vi "DHE_Macro.vi"(8 "error in (no error)":errorcluster, 10 "macro":string, 11 "fd":i32) -> (0 "error out":errorcluster, 2 "response":string)   [LabVIEW 2016]
panel:
  in  "refnum":refnum<vi>
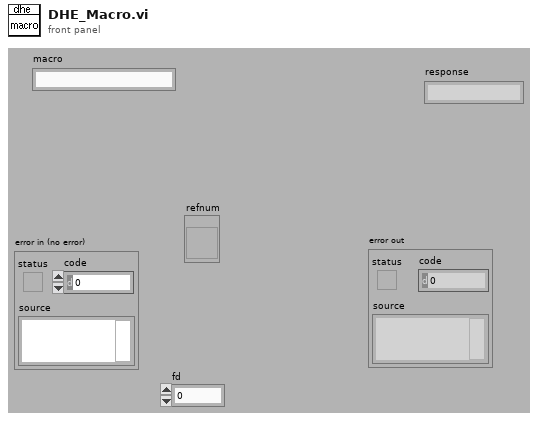
[diagram p1: front panel]
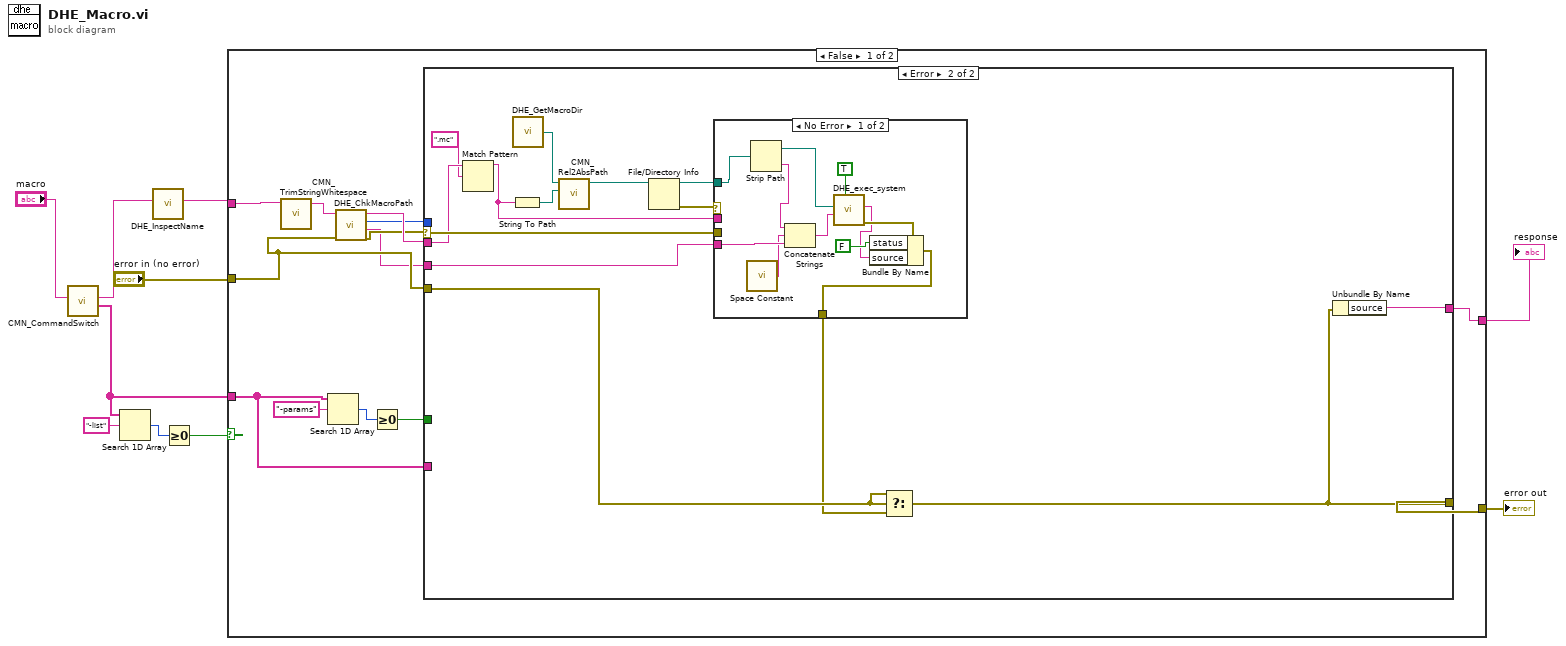
[diagram p0: block diagram]
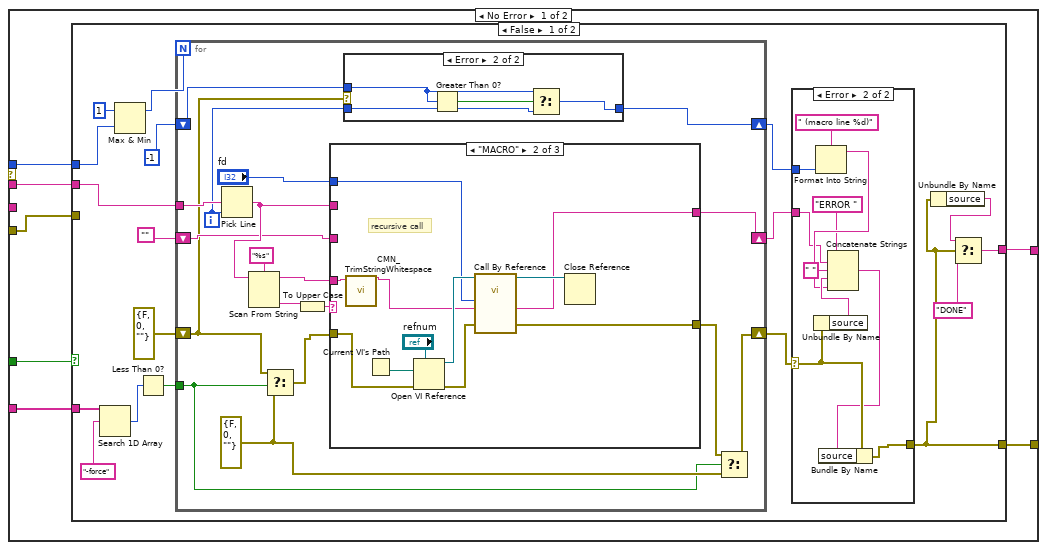
[diagram p2: hidden frame]
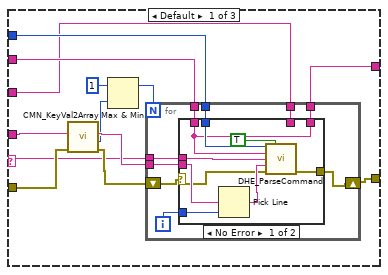
[diagram p4: hidden frame]
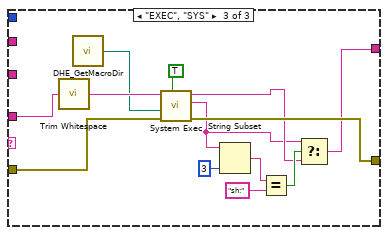
[diagram p6: hidden frame]
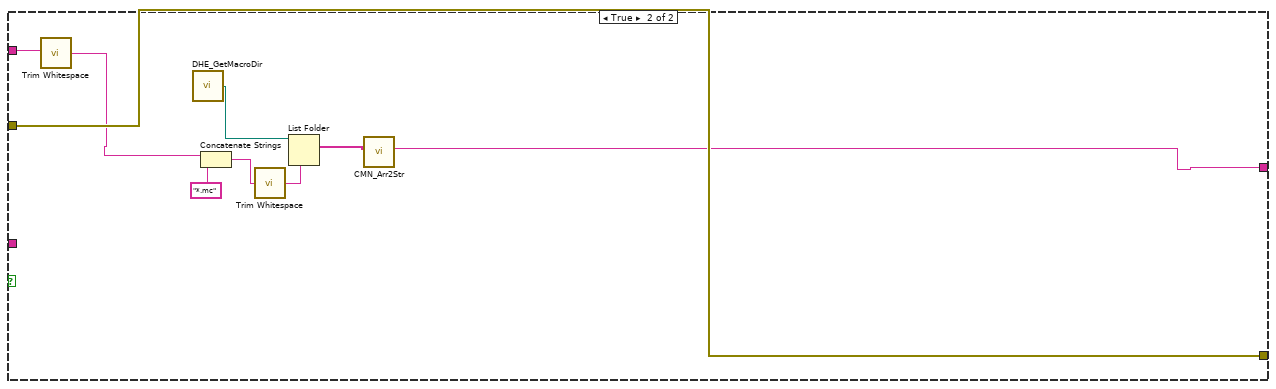
[diagram p10: hidden frame]
diagram:
  n1 = call "CMN_CommandSwitch.vi"("command in"="macro") -> ("swhitches"=w3:string[], "command out"=w2:string)  [unwired: 1 in, 8 out]
  n2 = Search 1D Array(1D array=w3, element="-list") -> (index of element=w8:i32)  [unwired: 1 out]
  n3 = call "DHE_InspectName.vi"("name in"=w2) -> ("name out"=w1:string)  [unwired: 10 out]
  n4 = Greater Or Equal To 0?(x=w8) -> (x >= 0?=w6:bool)
  n5 = case shown="False" w6 {
    tunnel: [w18 w174] -> w10
    tunnel: w1 -> [w20 w169]
    tunnel: "error in (no error)" -> [w19 w174]
    tunnel: [w14 w173] -> w5
    tunnel: w3 -> [w13 _]
    frame False {
      n6 = call "CMN_TrimStringWhitespace.vi"("string"=w20) -> ("trimmed string"=w12:string)  [unwired: 1 in, 8 out]
      n7 = Search 1D Array(1D array=w13, element="-params") -> (index of element=w16:i32)  [unwired: 1 out]
      n8 = call "DHE_ChkMacroPath.vi"("error in (no error)"=w19, "macro name"=w12) -> ("error out"=w22:errorcluster, "args"=w11:string, "number of lines"=w21:i32, "macro out"=w23:string)  [unwired: 6 out]
      n9 = Greater Or Equal To 0?(x=w16) -> (x >= 0?=w15:bool)
      n10 = case shown="Error" w22 {
        selector: w22 -> [_ w147]
        tunnel: [w27 w154] -> w18
        tunnel: w23 -> [w29 w144]
        tunnel: w21 -> [w30 _]
        tunnel: w19 -> [w25 w155]
        tunnel: w15 -> [w28 _]
        tunnel: [w26 w153] -> w14
        tunnel: w13 -> [w24 _]
        tunnel: w11 -> [_ w145]
        frame No Error {
          n11 = case shown="False" w28 {
            tunnel: w30 -> [w46 _]
            tunnel: w29 -> [w45 w141]
            tunnel: [w38 w140] -> w27
            tunnel: [w37 w141] -> w26
            tunnel: w25 -> [_ w140]
            tunnel: w24 -> [w34 _]
            frame False {
              n12 = Search 1D Array(1D array=w34, element="-force") -> (index of element=w32:i32)  [unwired: 1 out]
              n13 = Max & Min(x=1, y=w46) -> (max(x,y)=w47:i32)  [unwired: 1 out]
              n14 = Less Than 0?(x=w32) -> (x < 0?=w31:bool)
              n15 = for {
                N: w47 -> [_]
                shift-right: [w60] -> w42
                shift-left: errorcluster {"status"=FALSE, "code"=0, "source"=""} ("error out") -> [w65]
                tunnel: w45 -> [w74]
                shift-right: [w72] -> w41
                shift-left: -1 -> [w71]
                shift-right: [w68] -> w36
                shift-left: "" -> [w67]
                tunnel: w31 -> [w61]
                i -> [w73]
                w62 = errorcluster {"status"=FALSE, "code"=0, "source"=""} ("f")
                n16 = Pick Line(multi-line string=w74, line index=w73) -> (output string=w69:string)  [unwired: 1 out]
                n17 = Scan From String(format string="%s", input string=w69) -> (remaining string=w75:string, output 1=w76:string)  [unwired: 2 in, 3 out]
                n18 = Select(t=w65, s=w61, f=w62) -> (s? t:f=w64:errorcluster)
                n19 = To Upper Case(1:w76) -> (0:w66:string)
                n20 = case shown="\"MACRO\"" w66 {
                  selector: w66 -> [w83 _ _]
                  tunnel: w69 -> [w80 _ _]
                  tunnel: w75 -> [w84 w121 w132]
                  tunnel: w64 -> [w85 w114 w133]
                  tunnel: [w82 w116 w134] -> w63
                  tunnel: "fd" -> [w81 w115 _]
                  tunnel: [w79 w111 w124] -> w68
                  tunnel: w67 -> [w78 _ _]
                  frame Default {
                    n21 = call "CMN_KeyVal2Array.vi"("error in (no error)"=w85, "command in"=w84) -> ("error out"=w89:errorcluster, "number of commands"=w88:i32, "commands out"=w90:string)  [unwired: 1 in, 5 out]
                    n22 = Max & Min(x=1, y=w88) -> (max(x,y)=w86:i32)  [unwired: 1 out]
                    n23 = for {
                      N: w86 -> [_]
                      tunnel: w81 -> [w99]
                      tunnel: w80 -> [w98]
                      tunnel: w83 -> [w97]
                      tunnel: w90 -> [w94]
                      shift-right: [w96] -> w82
                      shift-left: w89 -> [w93]
                      tunnel: [w92] -> w79
                      tunnel: w78 -> [w91]
                      i -> [w95]
                      n24 = case shown="No Error" w93 {
                        selector: w93 -> [w102 w110]
                        tunnel: w99 -> [w108 _]
                        tunnel: w98 -> [w101 _]
                        tunnel: w97 -> [w107 _]
                        tunnel: [w106 w110] -> w96
                        tunnel: w95 -> [w105 _]
                        tunnel: w94 -> [w104 _]
                        tunnel: [w101 w109] -> w92
                        tunnel: w91 -> [_ w109]
                        frame No Error {
                          n25 = Pick Line(multi-line string=w104, line index=w105) -> (output string=w103:string)  [unwired: 1 out]
                          n26 = call "DHE_ParseCommand.vi"("fd"=w108, "Log"=TRUE, "command + args"=w101, "command"=w107, "arguments"=w103, "error in"=w102) -> ("error out"=w106:errorcluster)  [unwired: 1 in, 8 out]
                        }
                        frame Error {
                        }
                      }
                    }
                  }
                  frame "MACRO" {
                    # "recursive call"
                    n27 = call "CMN_TrimStringWhitespace.vi"("string"=w121) -> ("trimmed string"=w117:string)  [unwired: 1 in, 8 out]
                    n28 = Current VI's Path() -> (path=w119:path)
                    n29 = Open VI Reference(type specifier VI Refnum (for type only)="refnum", vi path=w119, error in (no error)=w114) -> (vi reference=w118:refnum<vi>, error out=w113:errorcluster)  [unwired: 3 out]
                    n30 = call-by-ref "?"(reference=w118, "error in (no error)"=w113, "macro"=w117, "fd"=w115) -> (reference out=w112:refnum<vi>, "error out"=w116:errorcluster, "response"=w111:string)  [unwired: 8 in, 1 out]
                    n31 = Close Reference(reference=w112) -> ()  [unwired: 1 in, 1 out]
                  }
                  frame "EXEC", "SYS" {
                    n32 = call <vilib>:"Trim Whitespace.vi"("string"=w132) -> ("trimmed string"=w131:string)  [unwired: 1 in]
                    n33 = call "DHE_GetMacroDir.vi"() -> ("DHE_MacroDir"=w129:path)  [unwired: 9 out]
                    n34 = call <vilib>:"System Exec.vi"("wait until completion? (T)"=TRUE, "error in (no error)"=w133, "working directory"=w129, "command line"=w131) -> ("error out"=w134:errorcluster, "standard error"=w122:string, "standard output"=w123:string)  [unwired: 2 in, 3 out]
                    n35 = String Subset(string=w122, length (rest)=3 ("length (rest)")) -> (substring=w125:string)  [unwired: 1 out]
                    n36 = Equal?(x=w125, y="sh:") -> (x = y?=w126:bool)
                    n37 = Select(t=w122, s=w126, f=w123) -> (s? t:f=w124:string)
                  }
                }
                n38 = case shown="Error" w65 {
                  tunnel: w73 -> [_ w137]
                  tunnel: [w135 w136] -> w72
                  tunnel: w71 -> [w135 w138]
                  frame No Error {
                  }
                  frame Error {
                    n39 = Greater Than 0?(x=w138) -> (x > 0?=w139:bool)
                    n40 = Select(t=w138, s=w139, f=w137) -> (s? t:f=w136:i32)
                  }
                }
                n41 = Select(t=w63, s=w61, f=w62) -> (s? t:f=w60:errorcluster)
              }
              n42 = case shown="Error" w42 {
                selector: w42 -> [w49 w58]
                tunnel: [w49 w57] -> w38
                tunnel: w41 -> [_ w55]
                tunnel: w36 -> [_ w51]
                frame No Error {
                }
                frame Error {
                  n43 = Unbundle By Name(w58) -> ("source"=w59:string)
                  n44 = Format Into String(format string=" (macro line %d)", w55) -> (resulting string=w53:string)  [unwired: 2 in, 1 out]
                  n45 = Concatenate Strings("ERROR " ("string"), w51, " " ("string"), w59, w53) -> (w56:string)
                  n46 = Bundle By Name(cluster=w58, "source"=w56) -> (w57:errorcluster)
                }
              }
              n47 = Unbundle By Name(w38) -> ("source"=w39:string)
              n48 = Select(t=w39, s=w38, f="DONE") -> (s? t:f=w37:string)
            }
            frame True {
            }
          }
        }
        frame Error {
          n49 = Match Pattern(string=w144, regular expression=".mc") -> (before substring=w142:string)  [unwired: 1 in, 3 out]
          n50 = String To Path(string=w142) -> (path=w149:path)
          n51 = call "DHE_GetMacroDir.vi"() -> ("DHE_MacroDir"=w150:path)  [unwired: 9 out]
          n52 = call "CMN_Rel2AbsPath.vi"("test path"=w149, "absolute path"=w150) -> ("output path"=w151:path)  [unwired: 1 in, 8 out]
          n53 = File/Directory Info(path=w151) -> (path out=w146:path, error out=w148:errorcluster)  [unwired: 1 in, 5 out]
          n54 = case shown="No Error" w148 {
            tunnel: [w160 w167] -> w152
            tunnel: w147 -> [_ w167]
            tunnel: w146 -> [w159 _]
            tunnel: w142 -> [_ _]
            tunnel: w145 -> [w165 _]
            frame No Error {
              n55 = call <vilib>:"Space Constant.vi"() -> ("String"=w157:string)
              n56 = Strip Path(path=w159) -> (stripped path=w158:path, name=w156:string)
              n57 = Concatenate Strings(w156, w157, w165) -> (w164:string)
              n58 = call "DHE_exec_system.vi"("wait until completion? (T)"=TRUE, "command line"=w164, "working directory"=w158) -> ("error out"=w163:errorcluster, "response"=w161:string)  [unwired: 7 in]
              n59 = Bundle By Name(cluster=w163, "status"=FALSE, "source"=w161) -> (w160:errorcluster)
            }
            frame Error {
            }
          }
          n60 = Select(t=w155, s=w155, f=w152) -> (s? t:f=w154:errorcluster)
          n61 = Unbundle By Name(w154) -> ("source"=w153:string)
        }
      }
    }
    frame True {
      n62 = call <vilib>:"Trim Whitespace.vi"("string"=w169) -> ("trimmed string"=w168:string)  [unwired: 1 in]
      n63 = call "DHE_GetMacroDir.vi"() -> ("DHE_MacroDir"=w176:path)  [unwired: 9 out]
      n64 = Concatenate Strings(w168, "*.mc" ("string")) -> (w171:string)
      n65 = call <vilib>:"Trim Whitespace.vi"("string"=w171) -> ("trimmed string"=w170:string)  [unwired: 1 in]
      n66 = List Folder(path=w176, pattern=w170) -> (filenames=w175:string[])  [unwired: 1 in, 4 out]
      n67 = call "CMN_Arr2Str.vi"("Array in"=w175) -> ("string out"=w173:string)  [unwired: 10 out]
    }
  }
  "error out" <- w10
  "response" <- w5
